vi "3D Omni Robot test.vi"() -> ()   [LabVIEW 2015]
doc: "This example shows how to use the Steering VIs to define and simulate a dynamic model of a three-wheeled omnidirectional robot on a smooth surface."
uses:
  Program Files (x86)/National Instruments/LabVIEW 2015/examples/robotics/Steering/3D Omni Robot/Robot Position.ctl
  <vilib>/robotics/Steering/Wheel/Wheel Parameters.ctl
  <vilib>/robotics/Steering/Wheel/Rotation Direction.ctl
  <vilib>/Simulation/Scripting/Companion Diagram/SimConfigNode/SimParams.ctl
  <vilib>/Simulation/Scripting/Companion Diagram/SimConfigNode/_simSolvers.ctl
  <vilib>/Simulation/Implementation/Shared/SIMSCR Execution Mode.ctl
  <vilib>/Platform/TimedLoop/XDataNode/timing_clust.ctl
  <vilib>/Platform/TimedLoop/XDataNode/nitl_modes.ctl
  <vilib>/Platform/TimedLoop/XDataNode/wakeup.ctl
  <vilib>/Simulation/Param Hierarchy/Typedefs/SIMPH Param Control Actions.ctl
  <vilib>/Simulation/Implementation/Shared/NILVSim_ParamChanged.vi
  <vilib>/Simulation/Implementation/Shared/NILVSim_FinishedLate.vi
  <vilib>/Simulation/Implementation/Shared/NILVSIM_BeginStep.vi
  <vilib>/Simulation/Utility/Implementation/SIM Halt.vi
  <vilib>/Simulation/Implementation/Shared/NILVSim_Manager.vi
  <vilib>/Utility/error.llb/Clear Errors.vi
  <vilib>/Simulation/Implementation/Shared/NILVSim_FinalizeModel.vi
  <vilib>/Analysis/coordinate.llb/2D Cartesian Coordinate Rotation.vi
  <vilib>/Analysis/coordinate.llb/2D Cartesian Coordinate Rotation (Scalar).vi
  <vilib>/robotics/Steering/Omnidirectional Wheel/Create Omnidirectional Wheel.vi
  <vilib>/robotics/Steering/Steering Frame/Create User Defined Steering Frame.vi
  <vilib>/Simulation/Implementation/Shared/SIM Unbundle Sim Info.vi
  <vilib>/Simulation/Implementation/Shared/SIMSH Read Queue.vi
  <vilib>/Simulation/Implementation/Shared/NILVSim_Initialize.vi
  <vilib>/Simulation/Utility/Implementation/NILVSim Get Time and IsAcceptedStep.vi
  <vilib>/Simulation/Implementation/Shared/NILVSim_GetModelError.vi
  <vilib>/Simulation/Implementation/Shared/SIM Bundle Sim Info.vi
  <vilib>/robotics/Steering/Steering Frame/Apply Steering Frame Velocity to Motors.vi
  <vilib>/robotics/Steering/Steering Frame/Get Steering Frame Velocity from Motors.vi
  <vilib>/Simulation/Scripting/Companion Diagram/SimConfigNode/SimDog.xnode
  Program Files (x86)/National Instruments/LabVIEW 2015/examples/robotics/Steering/3D Omni Robot/Omni Robot Model.vi
  <vilib>/Platform/TimedLoop/XDataNode/XDataNode.xnode
  <vilib>/Simulation/Implementation/XNodeFramework/SimXNode/SimX.xnode
  <vilib>/robotics/Steering/Steering Frame/NI_Robotics_Steering Frame.lvclass
  <vilib>/robotics/Steering/Wheel/NI_Robotics_Wheel.lvclass
  <vilib>/Platform/TimedLoop/XDataNode/XDNodeRunTimeDep.lvlib
  <vilib>/Simulation/Implementation/Shared/NI_SIM_Implementation.lvlib
  <vilib>/robotics/Steering/Omnidirectional Wheel/NI_Robotics_Omnidirectional Wheel.lvclass
panel:
  out "Waveform Chart 2":T1(graph)
  out "xy theta":T1(graph)
  in  "Velocity":T2(ring)
  out "motor states":dbl[](array[numeric]) format="%#.3f"
  in  "motor setpoints":dbl[](array[numeric])=[0.0, 0.0, 0.0] format="%#.3f"
  in  "reset":bool
  out "complete":bool
  in  "stop":bool
  out "robot position":T3 {"ccw wheel angles" format="%#.3f"; "global theta" format="%#.3f"; "global y" format="%#.3f"; "global x" format="%#.3f"}
  in  "Angular Velocity (rad/s)":dbl(slide) min=-7.0 max=7.0 scale=-7.0..7.0
  out "Angular Velocity Feedback":dbl(slide) scale=1.0..-1.0
  in  "Y Velocity (m/s)":dbl(slide) min=-100.0 max=100.0 scale=-100.0..100.0
  out "Y Velocity Feedback":dbl(slide) scale=-1.0..1.0
  in  "X Velocity (m/s)":dbl(slide) min=-100.0 max=100.0 scale=-100.0..100.0
  out "X Velocity Feedback":dbl(slide) scale=-1.0..1.0
  out "3D Picture":refnum<vi>(3d-picture)
  # "This VI simulates the steering of a three-wheeled omnidirectional robot on a smooth surface.\n\n1. Run the VI, then move the sliders to control the forward, lateral, and angular velocity components of the robot.\n\n2. Press the Reset Position button to move the robot back to its starting position."
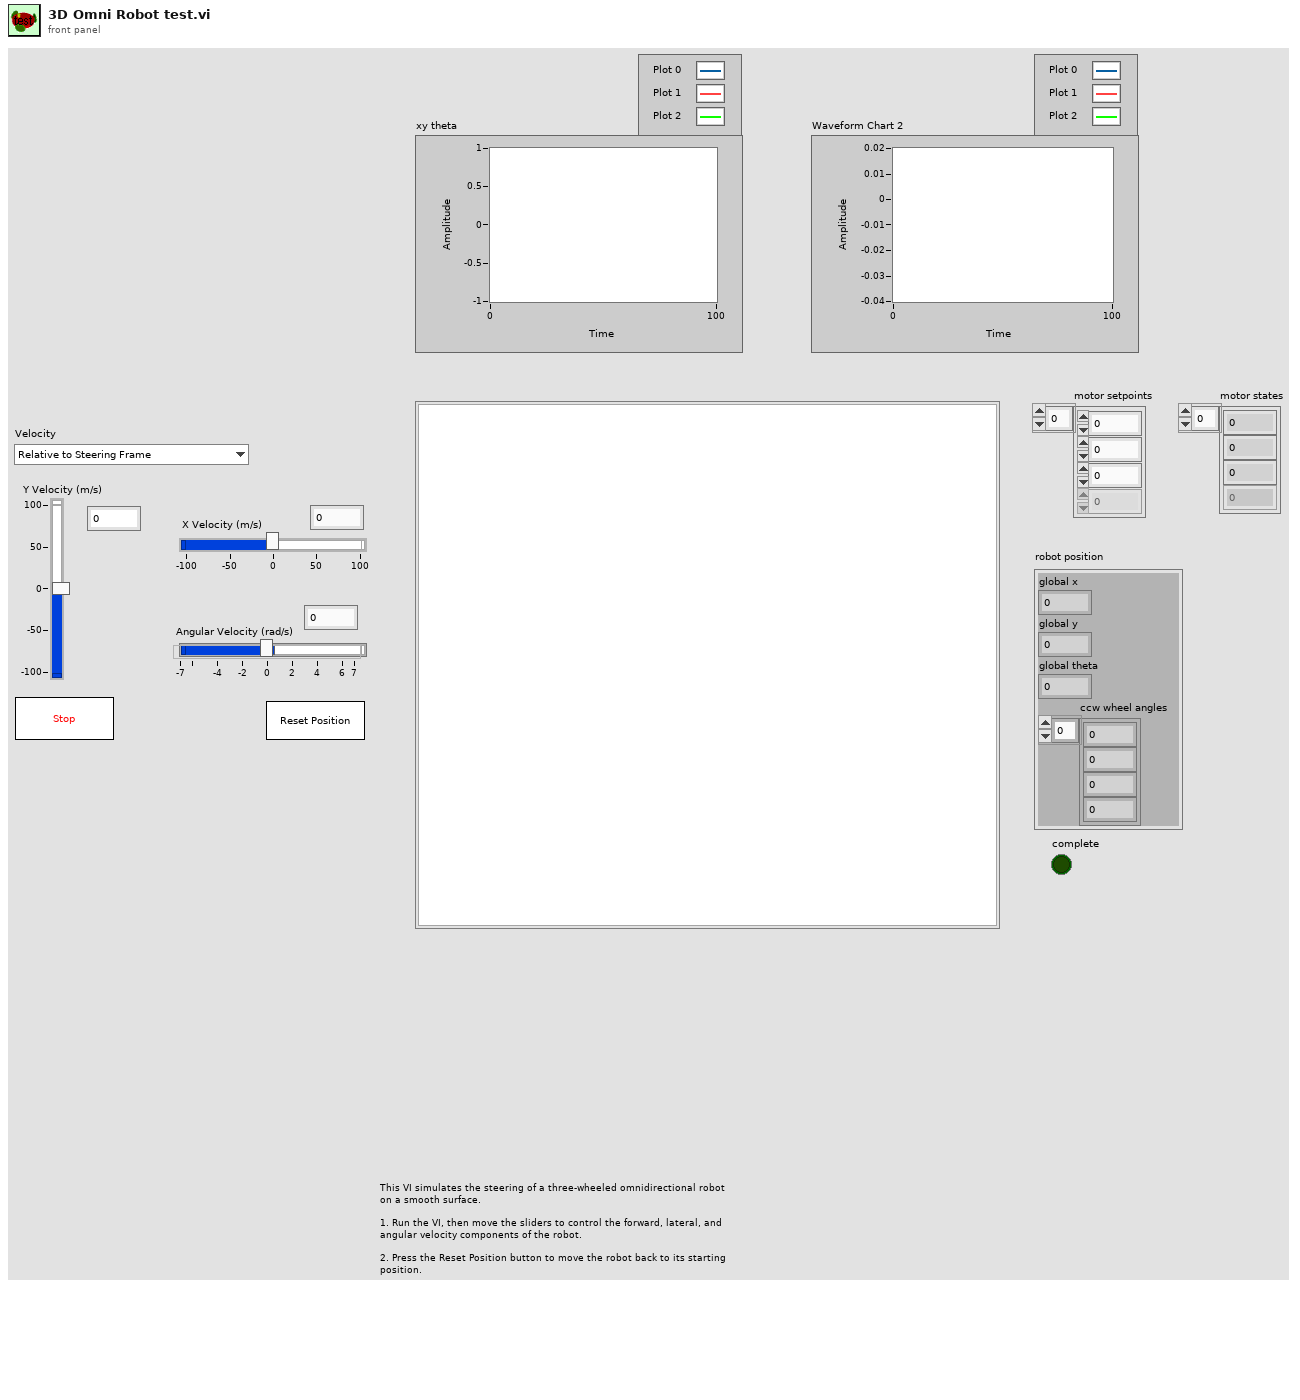
[diagram p1: front panel]
types:
  T1 = cluster{"motor states[0]":dbl, "motor states[1]":dbl, "motor states[2]":dbl, "motor states[3]":dbl, "motor states[4]":dbl, "motor states[5]":dbl, "motor states[6]":dbl, "motor states[7]":dbl, "motor states[8]":dbl}
  T2 = enum16{"Relative to Steering Frame", "Relative to Global Frame"}
  T3 = typedef "Robot Position.ctl" = cluster{"global x":dbl, "global y":dbl, "global theta":dbl, "ccw wheel angles":dbl[]}
  T4 = typedef "NI_Robotics_Wheel.lvclass/Rotation Direction.ctl" = u16
  T5 = typedef "NI_Robotics_Wheel.lvclass/Wheel Parameters.ctl" = cluster{"wheel radius":dbl, "gear ratio":dbl, "forward rotation direction":T4}
  T6 = cluster{"[0]":dbl, "[1]":dbl, "[2]":dbl, "[3]":dbl, "[4]":dbl, "[5]":dbl, "[6]":dbl, "[7]":dbl, "[8]":dbl}
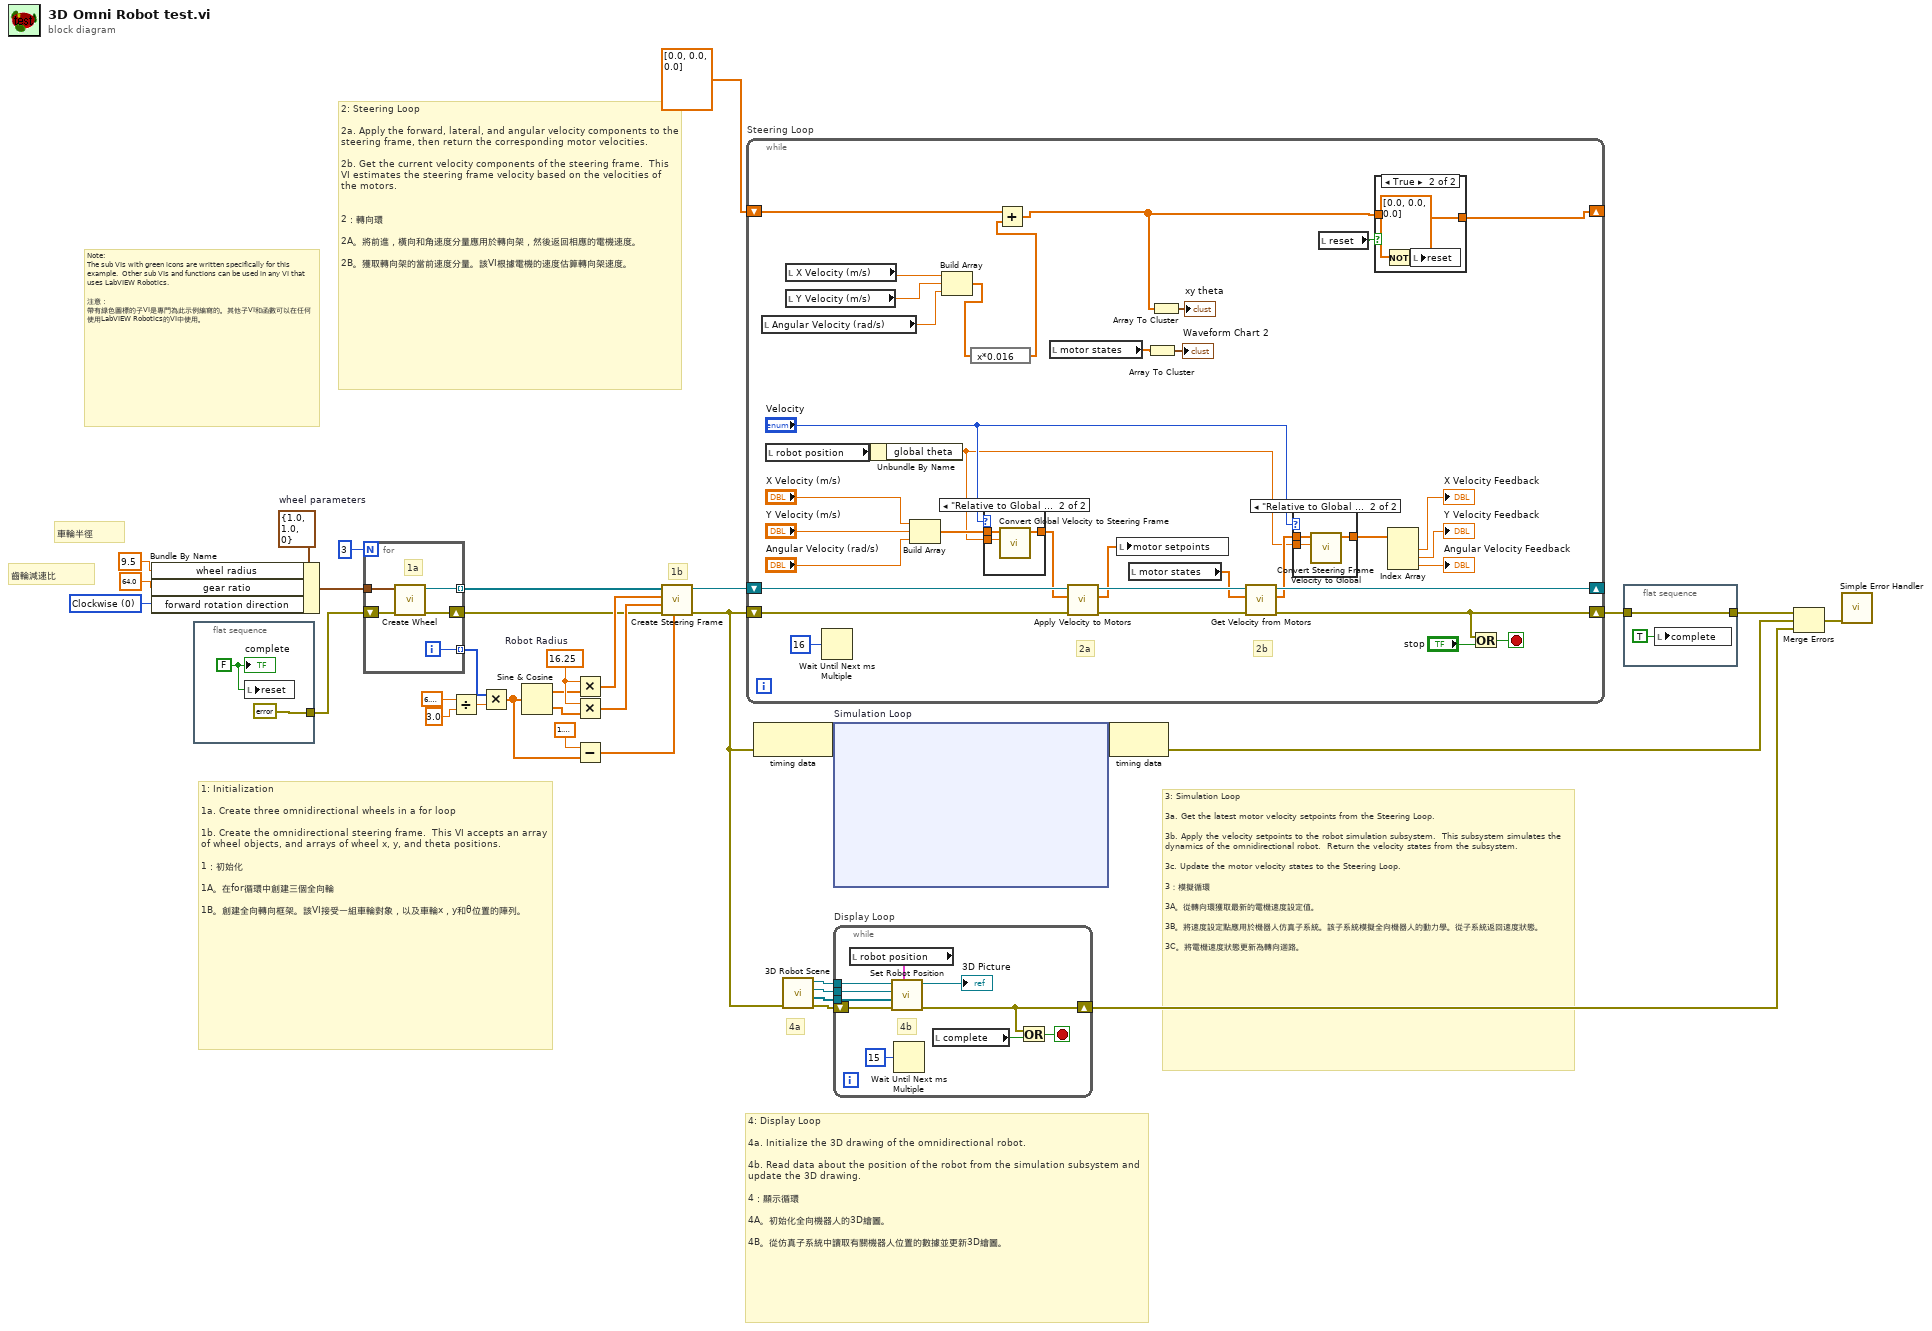
[diagram p0: block diagram]
diagram:
  w9 = T4 0 items=["Clockwise", "Counterclockwise"] ("forward rotation direction")
  w14 = 16.25  # Robot Radius
  w32 = T5 {"wheel radius"=1.0, "gear ratio"=1.0, "forward rotation direction"=0}  # wheel parameters
  # "齒輪減速比"
  # "車輪半徑"
  # "3: Simulation Loop\n\n3a. Get the latest motor velocity setpoints from the Steering Loop.\n\n3b. Apply the velocity setpoints to the robot simulation subsystem.  This subsystem simulates the dynamics of the omnidirectional robot.  Return the velocity states from the subsystem.\n\n3c. Update the motor velocity states to the Steering Loop.\n\n3：模擬循環\n\n3A。從轉向環獲取最新的電機速度設定值。\n\n3B。將速度設定點應用於機器人仿真子系統。該子系統模擬全向機器人的動力學。從子系統返回速度狀態。\n\n3C。將電機速度狀態更新為轉向迴路。"
  # "Note:\nThe sub VIs with green icons are written specifically for this example.  Other sub VIs and functions can be used in any VI that uses LabVIEW Robotics.\n\n注意：\n帶有綠色圖標的子VI是專門為此示例編寫的。其他子VI和函數可以在任何使用LabVIEW Robotics的VI中使用。"
  # "4a"
  # "4: Display Loop\n\n4a. Initialize the 3D drawing of the omnidirectional robot.\n\n4b. Read data about the position of the robot from the simulation subsystem and update the 3D drawing.\n\n4：顯示循環\n\n4A。初始化全向機器人的3D繪圖。\n\n4B。從仿真子系統中讀取有關機器人位置的數據並更新3D繪圖。"
  # "2: Steering Loop\n\n2a. Apply the forward, lateral, and angular velocity components to the steering frame, then return the corresponding motor velocities.\n\n2b. Get the current velocity components of the steering frame.  This VI estimates the steering frame velocity based on the velocities of the motors.\n\n\n2：轉向環\n\n2A。將前進，橫向和角速度分量應用於轉向架，然後返回相應的電機速度。\n\n2B。獲取轉向架的當前速度分量。該VI根據電機的速度估算轉向架速度。"
  # "1b"
  # "1: Initialization\n\n1a. Create three omnidirectional wheels in a for loop\n\n1b. Create the omnidirectional steering frame.  This VI accepts an array of wheel objects, and arrays of wheel x, y, and theta positions.\n\n1：初始化\n\n1A。在for循環中創建三個全向輪\n\n1B。創建全向轉向框架。該VI接受一組車輪對象，以及車輪x，y和θ位置的陣列。"
  n1 = Bundle By Name(cluster=w32, "wheel radius"=9.5, "gear ratio"=64.0, "forward rotation direction"=w9) -> (w29:T5)
  n2 = flat-sequence {
    tunnel: [errorcluster {"status"=FALSE, "code"=0, "source"=""} ("error out")] -> w24
    frame #0 {
      w36 = FALSE ("complete")
      n3 = local write "reset"(w36) -> ()
      "complete" <- w36
    }
  }
  n4 = for {
    N: 3 -> [_]
    shift-right: [w41] -> w6
    shift-left: w24 -> [w42]
    tunnel: [w40] -> w19 mode=indexing
    tunnel: w29 -> [w39]
    tunnel: [w38] -> w15 mode=indexing
    i -> [w38]
    # "1a"
    n5 = call-poly <vilib>:"Create Wheel.vi"("error in (no error)"=w42, "wheel parameters"=w39) -> ("error out"=w41:errorcluster, "omni wheel out"=w40:refnum<class "NI_Robotics_Omnidirectional Wheel.lvclass">)  [unwired: 8 in]
  }
  n6 = Divide(x=6.283185307179586, y=3.0) -> (x/y=w16:dbl)
  n7 = Multiply(x=w15, y=w16) -> (x*y=w4:dbl[])
  n8 = Sine & Cosine(0:w4) -> (1:w3:dbl[], 2:w2:dbl[])
  n9 = Multiply(x=w14, y=w3) -> (x*y=w13:dbl[])
  n10 = Multiply(x=w14, y=w2) -> (x*y=w12:dbl[])
  n11 = Subtract(x=1.5707963267948966, y=w4) -> (x-y=w10:dbl[])
  n12 = call-poly <vilib>:"Create Steering Frame.vi"("wheel frame angles (rad)"=w10, "error in (no error)"=w6, "wheel y positions"=w12, "wheel x positions"=w13, "wheels"=w19) -> ("error out"=w5:errorcluster, "steering frame out"=w33:refnum<class "NI_Robotics_Steering Frame.lvclass">)  [unwired: 5 in]
  n13 = while "Steering Loop" {
    shift-right: [w65] -> _
    shift-left: w33 -> [w68]
    shift-right: [w56] -> w25
    shift-left: w5 -> [w67]
    shift-right: [w45] -> _
    shift-left: dbl[] [0.0, 0.0, 0.0] -> [w54]
    stop <- w70 stop-if-true
    # "2b"
    # "2a"
    n14 = local read "Angular Velocity (rad/s)"() -> (w53:dbl)
    n15 = local read "robot position"() -> (w58:T3)
    n16 = local read "X Velocity (m/s)"() -> (w51:dbl)
    n17 = local read "Y Velocity (m/s)"() -> (w52:dbl)
    n18 = Wait Until Next ms Multiple(millisecond multiple=u32 16) -> ()  [unwired: 1 out]
    n19 = Unbundle By Name(w58) -> ("global theta"=w57:dbl)
    n20 = Build Array("X Velocity (m/s)", "Y Velocity (m/s)", "Angular Velocity (rad/s)") -> (w61:dbl[])
    n21 = Build Array(w51, w52, w53) -> (w44:dbl[])
    n22 = expression code="x*0.016"(w44) -> (w43:dbl[])
    n23 = case shown="\"Relative to Global Frame\"" "Velocity" {
      tunnel: w61 -> [w87 w90]
      tunnel: [w87 w89] -> w55
      tunnel: w57 -> [_ w88]
      frame "Relative to Steering Frame", Default {
      }
      frame "Relative to Global Frame" {
        n24 = call <vilib>:"Convert Global Velocity to Steering Frame.vi"("steering frame angle (rad)"=w88, "global velocity"=w90) -> ("steering frame velocity"=w89:dbl[])  [unwired: 9 in]
      }
    }
    n25 = Add(x=w54, y=w43) -> (x+y=w46:dbl[])
    n26 = local read "motor states"() -> (w49:dbl[])
    n27 = call-poly <vilib>:"Apply Velocity to Motors.vi"("error in (no error)"=w67, "steering frame velocity"=w55, "steering frame in"=w68) -> ("error out"=w66:errorcluster, "ccw motor velocity setpoints"=w64:dbl[], "steering frame out"=w69:refnum<class "NI_Robotics_Steering Frame.lvclass">)  [unwired: 4 in, 2 out]
    n28 = local write "motor setpoints"(w64) -> ()
    n29 = local read "motor states"() -> (w63:dbl[])
    n30 = Array To Cluster(array=w49) -> (cluster=→"Waveform Chart 2":T1)
    n31 = Array To Cluster(array=w46) -> (cluster=→"xy theta":T6)
    n32 = call-poly <vilib>:"Get Velocity from Motors.vi"("error in (no error)"=w66, "ccw motor velocity states"=w63, "steering frame in"=w69) -> ("error out"=w56:errorcluster, "estimated steering frame velocity"=w60:dbl[], "steering frame out"=w65:refnum<class "NI_Robotics_Steering Frame.lvclass">)  [unwired: 6 in]
    n33 = case shown="\"Relative to Global Frame\"" "Velocity" {
      tunnel: w60 -> [w83 w86]
      tunnel: [w83 w85] -> w59
      tunnel: w57 -> [_ w84]
      frame "Relative to Steering Frame", Default {
      }
      frame "Relative to Global Frame" {
        n34 = call <vilib>:"Convert Steering Frame Velocity to Global.vi"("steering frame angle (rad)"=w84, "steering frame velocity"=w86) -> ("global velocity"=w85:dbl[])  [unwired: 9 in]
      }
    }
    n35 = local read "reset"() -> (w47:bool)
    n36 = case shown="True" w47 {
      selector: w47 -> [_ w80]
      tunnel: w46 -> [w79 _]
      tunnel: [w79 dbl[] [0.0, 0.0, 0.0]] -> w45
      frame False {
      }
      frame True {
        n37 = Not(x=w80) -> (.not. x?=w81:bool)
        n38 = local write "reset"(w81) -> ()
      }
    }
    n39 = Index Array(array=w59) -> (element #1=→"X Velocity Feedback":dbl, element #2=→"Y Velocity Feedback":dbl, element #3=→"Angular Velocity Feedback":dbl)  [unwired: 3 in]
    n40 = Or(x=w56, y="stop") -> (x .or. y?=w70:bool)
  }
  n41 = node-c288(w5) -> (w35:variant)
  n42 = call "3D Robot Scene.vi"("error in (no error)"=w5) -> ("error out"=w21:errorcluster, "axles"=w26:refnum<vi>[], "robot"=w27:refnum<vi>, "scene"=w28:refnum<vi>)  [unwired: 7 in]
  n43 = node-c254 "Simulation Loop"(w35) -> (w34:variant)
  n44 = while "Display Loop" {
    tunnel: w28 -> [w94]
    tunnel: w27 -> [w95]
    tunnel: w26 -> [w96]
    shift-right: [w91] -> w20
    shift-left: w21 -> [w97]
    stop <- w92 stop-if-true
    # "4b"
    n45 = local read "robot position"() -> (w98:T3)
    n46 = call "Set Robot Position.vi"("robot position"=w98, "error in (no error)"=w97, "axles"=w96, "robot"=w95, "scene"=w94) -> ("error out"=w91:errorcluster, "scene out"=→"3D Picture":refnum<vi>)  [unwired: 5 in]
    n47 = Wait Until Next ms Multiple(millisecond multiple=u32 15) -> ()  [unwired: 1 out]
    n48 = local read "complete"() -> (w93:bool)
    n49 = Or(x=w91, y=w93) -> (x .or. y?=w92:bool)
  }
  n50 = node-c288(w34) -> (w7:errorcluster)
  n51 = flat-sequence {
    tunnel: w25 -> [w101]
    tunnel: [w101] -> w23
    frame #0 {
      n52 = local write "complete"(TRUE ("complete")) -> ()
    }
  }
  n53 = Merge Errors(w23, w7, w20) -> (w22:errorcluster)
  n54 = call <vilib>:"Simple Error Handler.vi"("error in (no error)"=w22) -> ()  [unwired: 4 in, 5 out]
